vi "Set ALEX.vi"(8 "error in (no error)":errorcluster, 9 "ALEX?":bool, 11 "Synchronization Device in":refnum<class "Synchronization Device.lvclass">) -> (0 "error out":errorcluster, 3 "Synchronization Device out":refnum<class "Synchronization Device.lvclass">)   [LabVIEW 2018, in "Synchronization Device.lvlib" / "Synchronization Device.lvclass"]
uses:
  Synchronization Device.lvclass
  Synchronization Device.lvclass/Synchronization Device.ctl
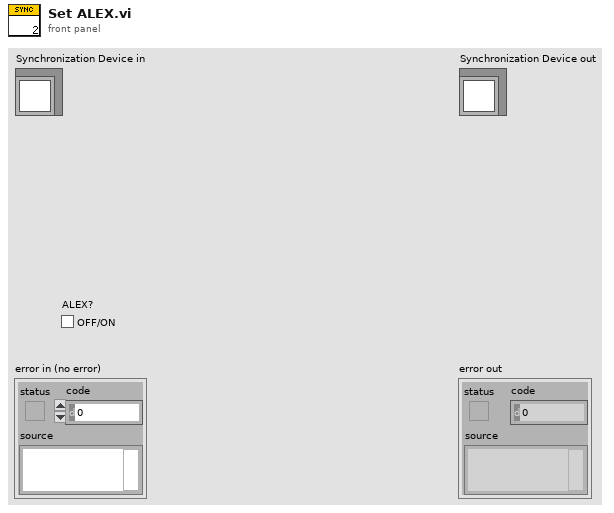
[diagram p1: front panel]
types:
  T1 = cluster{"Interval (ms)":dbl, "ALEX":bool, "Shutter Enable":bool[], "Stream":bool, "Duty Cycle":dbl}
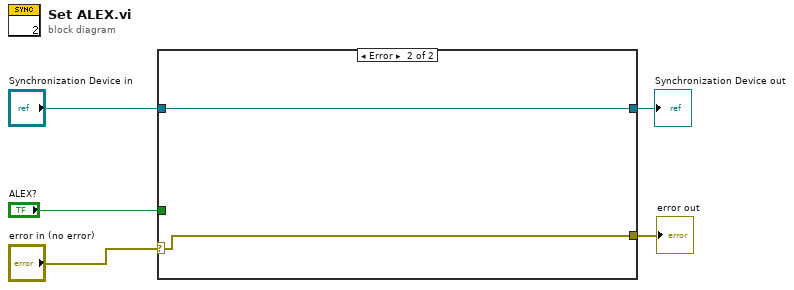
[diagram p0: block diagram]
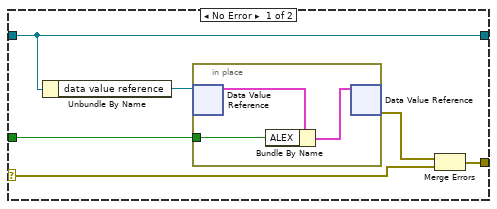
[diagram p2: hidden frame]
diagram:
  n1 = case shown="Error" "error in (no error)" {
    selector: "error in (no error)" -> [w6 w15]
    tunnel: [w10 w15] -> w5
    tunnel: [w11 w16] -> w4
    tunnel: "Synchronization Device in" -> [w11 w16]
    tunnel: "ALEX?" -> [w7 _]
    frame No Error {
      n2 = Unbundle By Name(w11) -> ("data value reference"=w9:refnum<data-value>)
      n3 = in-place {
        in-place-border: w7 -> [w12]
        n4 = in-place-dvr #1(w9) -> (w13:T1)  [unwired: 1 out]
        n5 = Bundle By Name(cluster=w13, "ALEX"=w12) -> (w14:T1)
        n6 = in-place-dvr #1(w14) -> (w8:errorcluster)  [unwired: 1 out]
      }
      n7 = Merge Errors(w8, w6) -> (w10:errorcluster)
    }
    frame Error {
    }
  }
  "error out" <- w5
  "Synchronization Device out" <- w4
